vi "Pre Build.vi"(0 "Compound_Installer In":refnum<class "Compound_Installer.lvclass">) -> (4 "Compound_Installer out":refnum<class "Compound_Installer.lvclass">)   [LabVIEW 2017, in "CL_G3_VIComponentBuilder.lvlib" / "Compound_Installer.lvclass"]
doc: "Executes any funtionality specified by the export before the export artifacts are created."
uses:
  Compound_Installer.lvclass
  C:/builds/Component BuilderBT/SrcDist/Exports/Exports/Export.lvclass
  Compound_Installer.lvclass/Compound_Installer.ctl
  Exports/Export.lvclass/Export.ctl
  Exports/Accessors/Read Export Artifacts for SCC.vi
  Exports/Accessors/Write Export Artifacts for SCC.vi
  Exports/Accessors/Write Export Operation Errors.vi
  Accessors/Read Sub Export Build Order.vi
  Exports/Accessors/Read Export Operation Errors.vi
  Exports/Export.lvclass
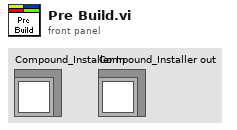
[diagram p1: front panel]
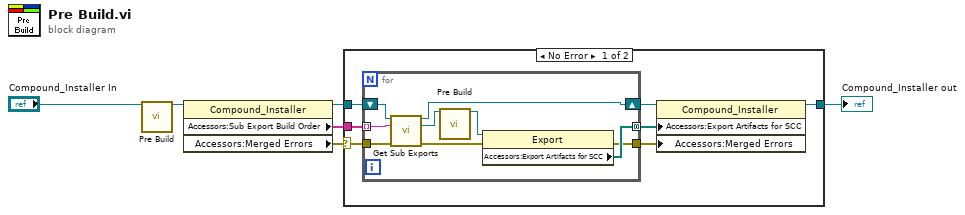
[diagram p0: block diagram]
diagram:
  n1 = call-parent "Pre Build.vi"("Export In"="Compound_Installer In") -> ("Export out"=w5:refnum<class "Compound_Installer.lvclass">)  [unwired: 14 in]
  n2 = property class="Compound_Installer"(reference=w5) -> (reference out=w4:refnum<class "Compound_Installer.lvclass">, "Accessors:Sub Export Build Order"=w3:string[], "Accessors:Merged Errors"=w1:errorcluster)  [unwired: 1 in, 1 out]
  n3 = case shown="No Error" w1 {
    selector: w1 -> [w12 _]
    tunnel: w4 -> [w13 w23]
    tunnel: w3 -> [w11 _]
    tunnel: [w8 w23] -> w2
    frame No Error {
      n4 = for {
        tunnel: w12 -> [w21]
        shift-right: [w14] -> w7
        shift-left: w13 -> [w22]
        tunnel: w11 -> [w19] mode=indexing
        tunnel: [w16] -> w10 mode=concatenating
        tunnel: [w15] -> w9
        n5 = call-dynamic "Get Sub Exports.vi"("NSIS_Installer in"=w22, "Sub Installer Name"=w19, "error in (no error)"=w21) -> ("NSIS_Installer out"=w14:refnum<class "Compound_Installer.lvclass">, "Export"=w18:refnum<class "Export.lvclass">, "error out"=w20:errorcluster)  [unwired: 9 in, 1 out]
        n6 = call-dynamic "Pre Build.vi"("Export In"=w18) -> ("Export out"=w17:refnum<class "Export.lvclass">)  [unwired: 14 in]
        n7 = property class="Export"(reference=w17, error in=w20) -> (error out=w15:errorcluster, "Accessors:Export Artifacts for SCC"=w16:path[])  [unwired: 1 out]
      }
      n8 = property class="Compound_Installer"(reference=w7, "Accessors:Export Artifacts for SCC"=w10, "Accessors:Merged Errors"=w9) -> (reference out=w8:refnum<class "Compound_Installer.lvclass">)  [unwired: 1 in, 1 out]
    }
    frame Error {
    }
  }
  "Compound_Installer out" <- w2
